vi "3.11-Get Parabolic Constants.vi"(2 "Number of affected points (z)":dbl, 3 "Scaled Magnitude":dbl) -> (0 "Graph scale factor (b)":dbl, 1 "parabolic constant (c)":dbl)   [LabVIEW 2011]
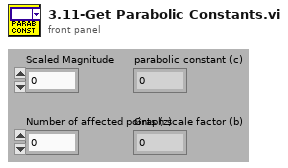
[diagram p1: front panel]
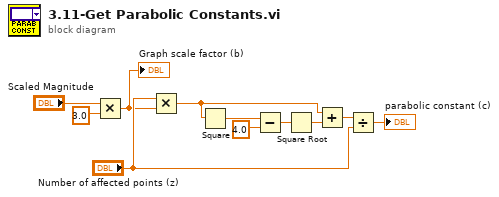
[diagram p0: block diagram]
diagram:
  n1 = Multiply(x="Scaled Magnitude", y=3.0) -> (x*y=w10:dbl)
  "Graph scale factor (b)" <- w10
  n2 = Multiply(x="Number of affected points (z)", y=w10) -> (x*y=w3:dbl)
  n3 = Square(x=w3) -> (x^2=w5:dbl)
  n4 = Subtract(x=w5, y=4.0) -> (x-y=w6:dbl)
  n5 = Square Root(x=w6) -> (sqrt(x)=w4:dbl)
  n6 = Add(x=w3, y=w4) -> (x+y=w8:dbl)
  n7 = Divide(x=w8, y="Number of affected points (z)") -> (x/y=→"parabolic constant (c)":dbl)
